vi "SSC Digital Configure Time Set Compare Edge.vi"(0 "Digital SSC in":T1[](array[typedef]), 5 "time set":string caption="Time Set", 7 "Compare Strobe (s)":dbl, 11 "error in":errorcluster) -> (4 "Digital SSC out":T1[](array[typedef]), 15 "error out":errorcluster)   [LabVIEW 2019]
doc: "Configures the strobe edge time for the specified pins. Use this function to modify time set values after applying a timing sheet with the niDigital Apply Levels and Timing VI, or to create time sets programmatically without the use of timing sheets. This function does not modify the timing sheet file or the timing sheet contents that will be used in future calls to niDigital Apply Levels and Timing; it only affects the values of the current timing context."
uses:
  SSC Digital.ctl
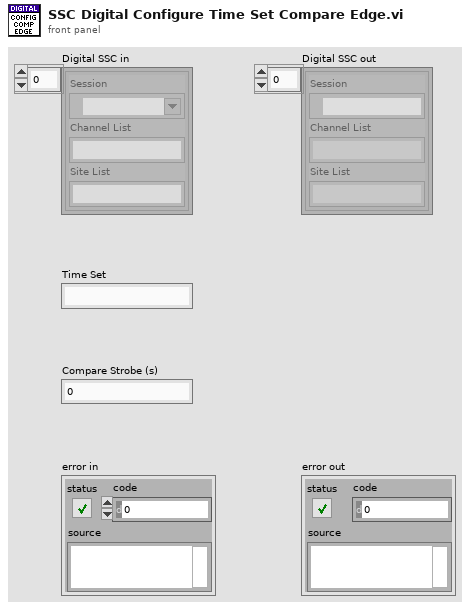
[diagram p1: front panel]
types:
  T1 = typedef "SSC Digital.ctl" = cluster{"Session":refnum<k15>, "Channel List":string, "Site List":string}
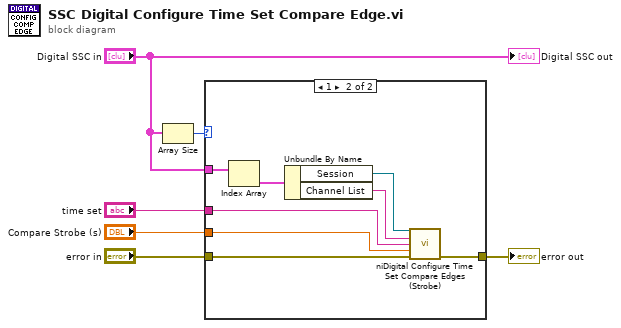
[diagram p0: block diagram]
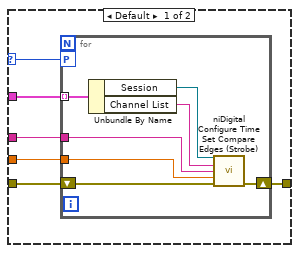
[diagram p2: hidden frame]
diagram:
  n1 = Array Size(array="Digital SSC in") -> (size(s)=w4:i32)
  n2 = case shown="1" w4 {
    selector: w4 -> [w12 _]
    tunnel: "error in" -> [w10 w27]
    tunnel: [w7 w26] -> w5
    tunnel: "Digital SSC in" -> [w11 w25]
    tunnel: "Compare Strobe (s)" -> [w8 w21]
    tunnel: "time set" -> [w9 w20]
    frame Default {
      n3 = for {
        workers-P: w12 -> [_]
        tunnel: w11 -> [w17] mode=indexing
        tunnel: w9 -> [w14]
        tunnel: w8 -> [w13]
        shift-right: [w18] -> w7
        shift-left: w10 -> [w19]
        n4 = Unbundle By Name(w17) -> ("Session"=w16:refnum<k15>, "Channel List"=w15:string)
        n5 = call <instrlib>:"niDigital Configure Time Set Compare Edges (Strobe).vi"("instrument handle"=w16, "pin list"=w15, "edge set"=w14, "compare strobe (s)"=w13, "error in"=w19) -> ("error out"=w18:errorcluster)  [unwired: 9 in, 1 out]
      }
    }
    frame 1 {
      n6 = Index Array(array=w25) -> (element=w22:T1)  [unwired: 1 in]
      n7 = Unbundle By Name(w22) -> ("Session"=w24:refnum<k15>, "Channel List"=w23:string)
      n8 = call <instrlib>:"niDigital Configure Time Set Compare Edges (Strobe).vi"("instrument handle"=w24, "pin list"=w23, "edge set"=w20, "compare strobe (s)"=w21, "error in"=w27) -> ("error out"=w26:errorcluster)  [unwired: 9 in, 1 out]
    }
  }
  "error out" <- w5
  "Digital SSC out" <- "Digital SSC in"
